vi "Error Cluster Descriptions Updater.vi"   [LabVIEW 2017]
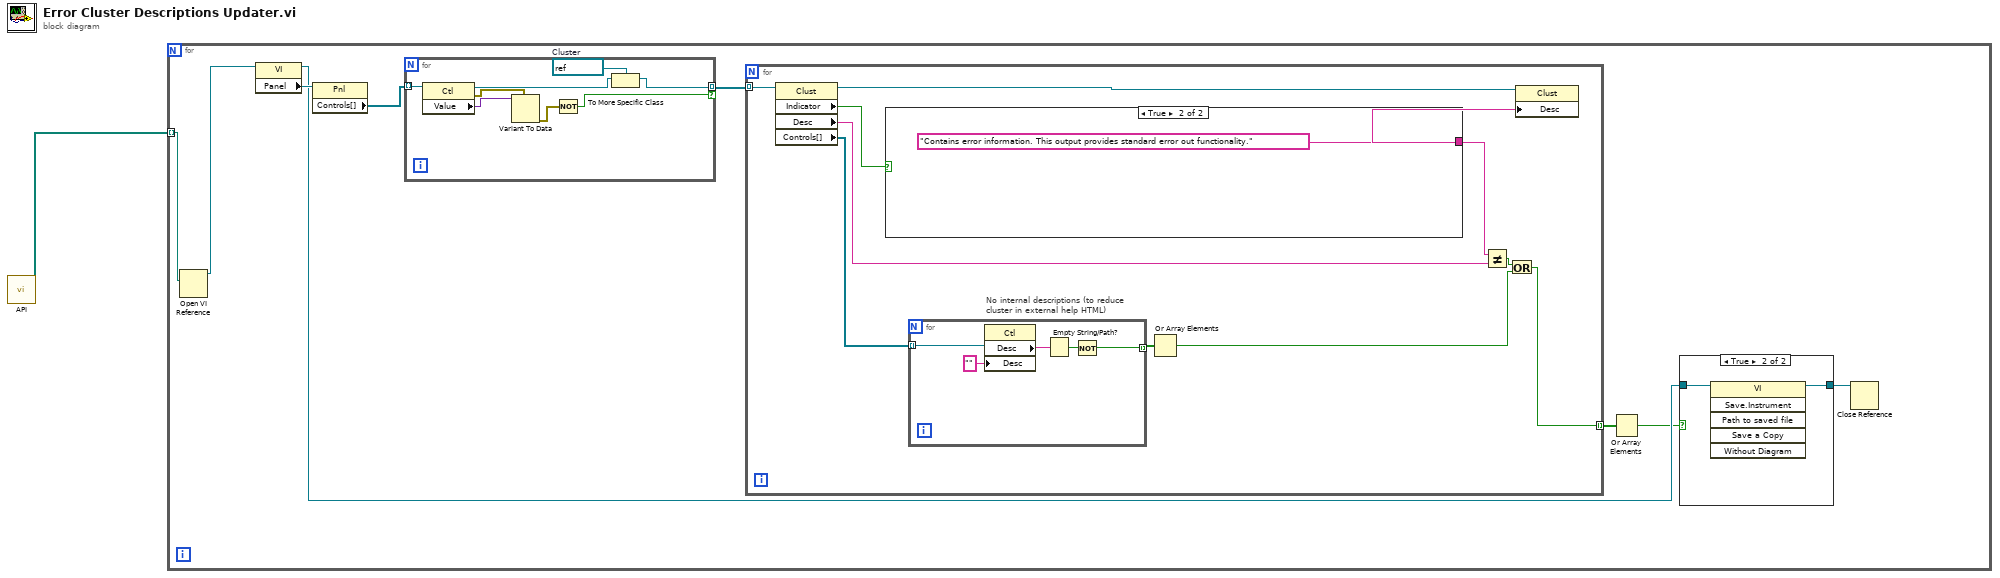
[diagram p0: block diagram]
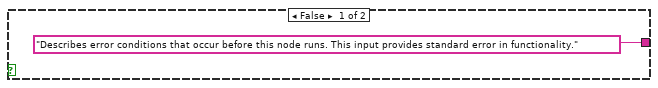
[diagram p2: hidden frame]
diagram:
  n1 = call "API.vi"() -> ("API"=w1:path[])  [unwired: 9 in, 2 out]
  n2 = for {
    tunnel: w1 -> [w9] mode=indexing
    n3 = Open VI Reference(vi path=w9) -> (vi reference=w8:refnum<vi>)  [unwired: 5 in, 1 out]
    n4 = property class="VI"(reference=w8) -> (reference out=w7:refnum<vi>, "Panel"=w10:refnum<vi>)  [unwired: 1 in, 1 out]
    n5 = property class="Pnl"(reference=w10) -> ("Controls[]"=w5:refnum<vi>[])  [unwired: 1 in, 2 out]
    n6 = for {
      tunnel: w5 -> [w35] mode=indexing
      tunnel: [w29] -> w4 mode=indexing if=w31
      w28 = refnum<vi> refnum  # Cluster
      n7 = property class="Ctl"(reference=w35) -> (reference out=w30:refnum<vi>, error out=w33:errorcluster, "Value"=w34:variant)  [unwired: 1 in]
      n8 = Variant To Data(type=w33, Variant=w34) -> (error out=w32:errorcluster)  [unwired: 1 in, 1 out]
      n9 = Not(x=w32) -> (.not. x?=w31:bool)
      n10 = To More Specific Class(target class=w28, reference=w30) -> (specific class reference=w29:refnum<vi>)  [unwired: 1 in, 1 out]
    }
    n11 = for {
      tunnel: w4 -> [w20] mode=indexing
      tunnel: [w11] -> w3 mode=indexing
      n12 = property class="Clust"(reference=w20) -> (reference out=w19:refnum<vi>, "Indicator"=w17:bool, "Desc"=w15:string, "Controls[]"=w18:refnum<vi>[])  [unwired: 1 in, 1 out]
      n13 = case shown="True" w17 {
        tunnel: ["Describes error conditions that occur before this node runs. This input provides standard error in functionality." "Contains error information. This output provides standard error out functionality."] -> w16
        frame False {
        }
        frame True {
        }
      }
      n14 = for "No internal descriptions (to reduce \ncluster in external help HTML)" {
        tunnel: w18 -> [w27] mode=indexing
        tunnel: [w23] -> w14 mode=indexing
        n15 = property class="Ctl"(reference=w27, "Desc"="" ("Description")) -> ("Desc"=w25:string)  [unwired: 1 in, 2 out]
        n16 = Empty String/Path?(string/path=w25) -> (empty?=w24:bool)
        n17 = Not(x=w24) -> (.not. x?=w23:bool)
      }
      n18 = Or Array Elements(Boolean array=w14) -> (logical OR=w12:bool)
      n19 = Not Equal?(x=w16, y=w15) -> (x != y?=w13:bool)
      n20 = Or(x=w13, y=w12) -> (x .or. y?=w11:bool)
      n21 = property class="Clust"(reference=w19, "Desc"=w16) -> ()  [unwired: 1 in, 2 out]
    }
    n22 = Or Array Elements(Boolean array=w3) -> (logical OR=w2:bool)
    n23 = case shown="True" w2 {
      tunnel: w7 -> [w36 w38]
      tunnel: [w36 w37] -> w6
      frame False {
      }
      frame True {
        n24 = invoke class="VI" method="Save.Instrument"(reference=w38) -> (reference out=w37:refnum<vi>)  [unwired: 5 in, 5 out]
      }
    }
    n25 = Close Reference(reference=w6) -> ()  [unwired: 1 in, 1 out]
  }
